vi "测量数据解析.vi"(11 "完整输入":string="\u0001\u0003\u0004\u0014\u0000\u0000\u0000ÿÃ") -> (0 "CRC？":bool, 2 "探头号":i32, 3 "测量值":dbl)   [LabVIEW 2017]
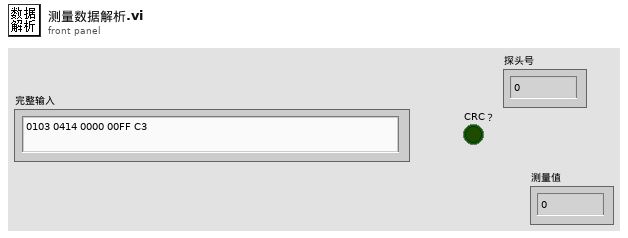
[diagram p1: front panel]
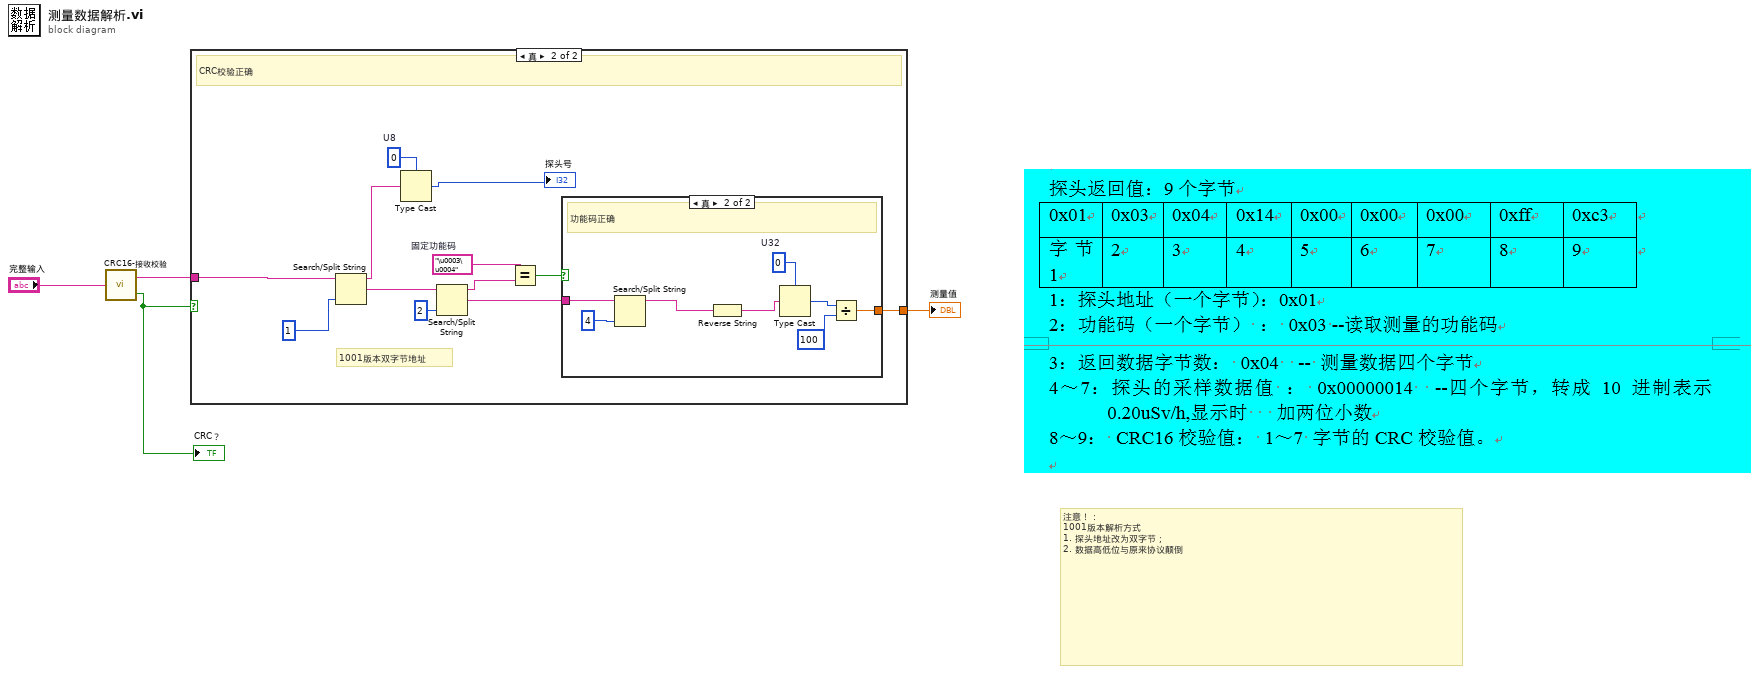
[diagram p0: block diagram]
diagram:
  # "注意！：\n1001版本解析方式\n1. 探头地址改为双字节；\n2. 数据高低位与原来协议颠倒"
  n1 = call "CRC16-接收校验.vi"("读取缓冲区"="完整输入") -> ("净数据"=w3:string, "CRC？"=w2:bool)
  "CRC？" <- w2
  n2 = case shown="真" w2 {
    tunnel: w3 -> [_ w11]
    tunnel: [_ w14] -> w1
    frame False {
    }
    frame True {
      w5 = u8 0  # U8
      w12 = "\u0003\u0004"  # 固定功能码
      # "1001版本双字节地址"
      # "CRC校验正确"
      n3 = Search/Split String(string=w11, offset (0)=1 ("偏移量(0)")) -> (substring before match=w7:string, match + rest of string=w10:string)  [unwired: 1 in, 1 out]
      n4 = Type Cast(type=w5, x=w7) -> (*(type *) &x=→"探头号":u8)
      n5 = Search/Split String(string=w10, offset (0)=2 ("偏移量(0)")) -> (substring before match=w13:string, match + rest of string=w15:string)  [unwired: 1 in, 1 out]
      n6 = Equal?(x=w12, y=w13) -> (x = y?=w9:bool)
      n7 = case shown="真" w9 {
        tunnel: w15 -> [_ w24]
        tunnel: [_ w19] -> w14
        frame False {
        }
        frame True {
          w22 = u32 0  # U32
          # "功能码正确"
          n8 = Search/Split String(string=w24, offset (0)=4 ("偏移量(0)")) -> (substring before match=w18:string)  [unwired: 1 in, 2 out]
          n9 = Reverse String(1:w18) -> (0:w17:string)
          n10 = Type Cast(type=w22, x=w17) -> (*(type *) &x=w21:u32)
          n11 = Divide(x=w21, y=u32 100) -> (x/y=w19:dbl)
        }
      }
    }
  }
  "测量值" <- w1
